vi "Wrapper.vi"(0 "measurement configuration":T1={"Calculate Analysis?"=TRUE, "Current Setpoint"=1.2, "Voltage Setpoint"=0.0, "Physical Channel"="Lorem ipsum dolor sit"}, 5 "Physical Channel":tag="PowerModule/power", 11 "error in":errorcluster) -> (4 "measurement results":T2, 15 "error out":errorcluster)   [LabVIEW 2021, in "Z Power Module.lvlib"]
uses:
  Z Power Module.lvlib
  Measurement Results.ctl
  Measurement Configuration.ctl
  MeasurementCore/Power Measurement/Z Power Module Main Library.lvlib
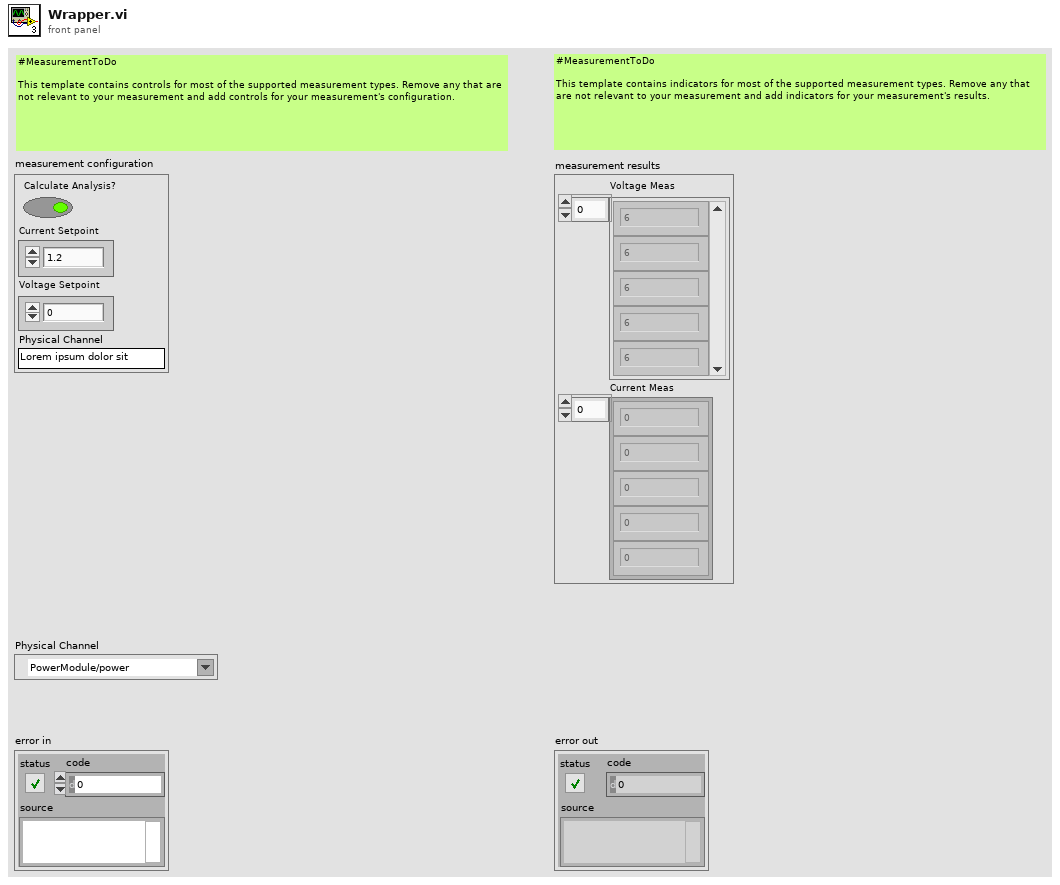
[diagram p1: front panel]
types:
  T1 = typedef "Z Power Module.lvlib/Measurement Configuration.ctl" = cluster{"Calculate Analysis?":bool, "Current Setpoint":dbl, "Voltage Setpoint":dbl, "Physical Channel":string}
  T2 = typedef "Z Power Module.lvlib/Measurement Results.ctl" = cluster{"Voltage Meas":dbl[], "Current Meas":dbl[]}
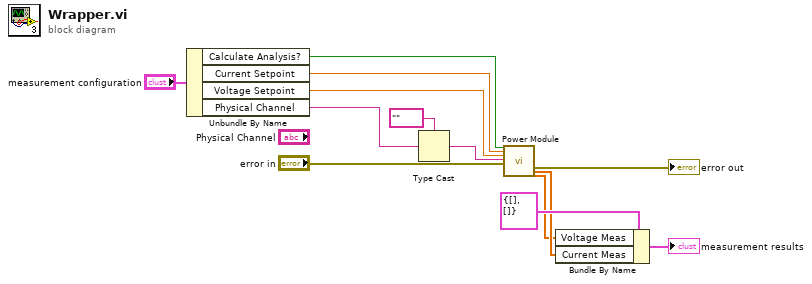
[diagram p0: block diagram]
diagram:
  n1 = Unbundle By Name("measurement configuration") -> ("Calculate Analysis?"=w8:bool, "Current Setpoint"=w7:dbl, "Voltage Setpoint"=w6:dbl, "Physical Channel"=w2:string)
  n2 = Type Cast(type=tag "" ("Physical Channel"), x=w2) -> (*(type *) &x=w1:tag)
  n3 = call "Power Module.vi"("Calculate Analysis?"=w8, "Current Setpoint"=w7, "Voltage Setpoint"=w6, "Physical Channel"=w1, "error in"="error in") -> ("error out"=→"error out":errorcluster, "Current Meas"=w11:dbl[], "Voltage Meas"=w10:dbl[])  [unwired: 20 in]
  n4 = Bundle By Name(cluster=T2 {"Voltage Meas"=[], "Current Meas"=[]} ("measurement results"), "Voltage Meas"=w10, "Current Meas"=w11) -> (→"measurement results":T2)
